vi "Angle Processing Unit.vi"(7 "settings.<user name>":T4, 8 "register bus":T2={"Speed"="Speed", "Crank Angle"="Crank Angle", "Cycle Angle"="Cycle Angle", "Crank Count"="Crank Count", "Cycle Count"="Cycle Count", "1.25 MHz Counter"="1.25 MHz Counter", "Crank Rollover"="Crank Rollover", "Cycle Rollover"="Cycle Rollover", "shared settings"={"start"=0.0, "stuck limit"=0.0}} {"shared settings"."start" format="%#.15g"}, 11 "input.<user name>":T1={"desired speed"=0.0, "reset"=TRUE}) -> (3 "output.<user name>":T5)   [LabVIEW 2015, in "Engine Simulation Toolkit.lvlib" / "APU.lvlib"]
doc: "Simulates a rotating engine with speed and (optionally) acceleration and publishes crank and cycle positions to the register bus. <b> This VI should be in an SCTL</b>\n\n<b>settings.<user name></b> - settings for the component. NI VeriStand will set these values. Create a control for this input. Replace <user name> with the name you wish this component to display as inside NI VeriStand. Make this name consistent for all controls, indicators, for all VIs of this component.\n<b>input.<user name></b> - input for the component. NI VeriStand will set these values. Create a control for this input. Replace <user name> with the name you wish this component to display as inside NI VeriStand. Make this name consistent for all controls, indicators, for all VIs of this component.\n<b>register bus</b> - connect this input to the output of the initialize APU VI. This contains references to APU state variables like position and speed.\n\n<b>output.<user name></b> - output for the component. NI VeriStand will read these values. Create an indicator for this output. Replace <user name> with the name you wish this component to display as inside NI VeriStand. Make this name consistent for all controls, indicators, for all VIs of this component."
uses:
  APU.lvlib
  Output.ctl
  Settings.ctl
  Register Bus.ctl
  Shared Settings.ctl
  Input.ctl
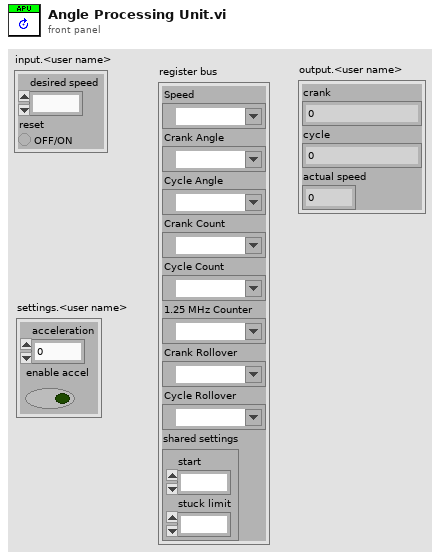
[diagram p1: front panel]
types:
  T1 = typedef "Engine Simulation Toolkit.lvlib/APU.lvlib/Input.ctl" = cluster{"desired speed":fxp<+/-,23,2>, "reset":bool}
  T2 = typedef "Engine Simulation Toolkit.lvlib/APU.lvlib/Register Bus.ctl" = cluster{"Speed":refnum<k21>, "Crank Angle":refnum<k21>, "Cycle Angle":refnum<k21>, "Crank Count":refnum<k21>, "Cycle Count":refnum<k21>, "1.25 MHz Counter":refnum<k21>, "Crank Rollover":refnum<k21>, "Cycle Rollover":refnum<k21>, "shared settings":T3}
  T3 = typedef "Engine Simulation Toolkit.lvlib/APU.lvlib/Shared Settings.ctl" = cluster{"start":fxp<+,17,17>, "stuck limit":fxp<+,18,18>}
  T4 = typedef "Engine Simulation Toolkit.lvlib/APU.lvlib/Settings.ctl" = cluster{"acceleration":fxp<+,18,-20>, "enable accel":bool}
  T5 = typedef "Engine Simulation Toolkit.lvlib/APU.lvlib/Output.ctl" = cluster{"crank":u16, "cycle":u16, "actual speed":fxp<+/-,23,2>}
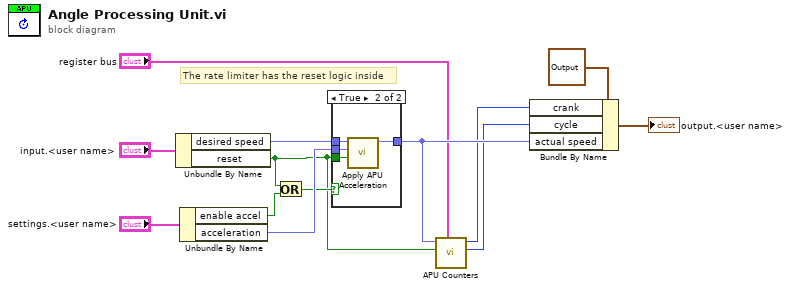
[diagram p0: block diagram]
diagram:
  # "The rate limiter has the reset logic inside"
  n1 = Unbundle By Name("input.<user name>") -> ("desired speed"=w5:fxp<+/-,23,2>, "reset"=w1:bool)
  n2 = Unbundle By Name("settings.<user name>") -> ("enable accel"=w3:bool, "acceleration"=w10:fxp<+,18,-20>)
  n3 = Or(x=w1, y=w3) -> (x .or. y?=w2:bool)
  n4 = case shown="True" w2 {
    tunnel: w10 -> [_ w18]
    tunnel: [w14 w17] -> w9
    tunnel: w5 -> [w14 w16]
    tunnel: w1 -> [_ w15]
    frame False {
    }
    frame True {
      n5 = call "Apply APU Acceleration.vi"("reset"=w15, "acceleration"=w18, "desired speed"=w16) -> ("actual speed"=w17:fxp<+/-,23,2>)  [unwired: 8 in]
    }
  }
  n6 = call "APU Counters.vi"("register bus"="register bus", "reset"=w1, "actual speed"=w9) -> ("cycle angle"=w8:u16, "crank angle"=w7:u16)  [unwired: 7 in]
  n7 = Bundle By Name(cluster=T5 {"crank"=0, "cycle"=0, "actual speed"=0.0} ("APU output v1.0.0"), "crank"=w7, "cycle"=w8, "actual speed"=w9) -> (→"output.<user name>":T5)
